vi "raise_any_errors.vi"(8 "error in (no error)":errorcluster, 11 "Request in":refnum<class "Request.lvclass">) -> (0 "error out":errorcluster, 3 "Request out":refnum<class "Request.lvclass">)   [LabVIEW 2020, in "reqwest.lvlib" / "Request.lvclass"]
uses:
  Request.lvclass
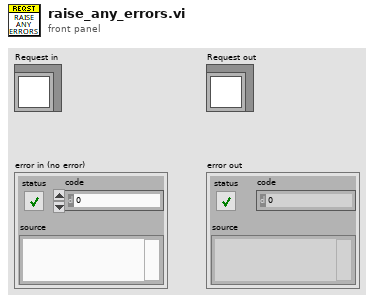
[diagram p1: front panel]
types:
  T1 = typedef "reqwest.lvlib/Request.lvclass/reqwest_error_kind_enum.ctl" = enum16{"none", "timeout", "connection", "redirect", "invalid_status", "body", "decode", "builder", "request", "file_system", "unknown"}
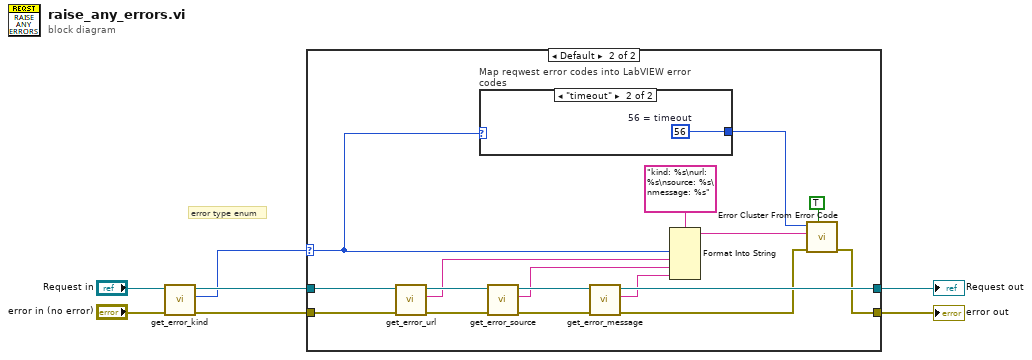
[diagram p0: block diagram]
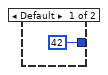
[diagram p3: hidden frame]
diagram:
  # "error type enum"
  n1 = call "get_error_kind.vi"("error in (no error)"="error in (no error)", "Request in"="Request in") -> ("error out"=w2:errorcluster, "error_kind"=w1:T1, "Request out"=w3:refnum<class "Request.lvclass">)  [unwired: 7 in]
  n2 = case shown="Default" w1 {
    selector: w1 -> [_ w10]
    tunnel: [w9 w26] -> w5
    tunnel: [w8 w25] -> w4
    tunnel: w3 -> [w9 w19]
    tunnel: w2 -> [w8 w18]
    frame "none" {
    }
    frame Default {
      n3 = call "get_error_url.vi"("error in (no error)"=w18, "Request in"=w19) -> ("error out"=w16:errorcluster, "error_url"=w15:string, "Request in"=w17:refnum<class "Request.lvclass">)  [unwired: 7 in]
      n4 = case "Map reqwest error codes into LabVIEW error codes" shown="\"timeout\"" w10 {
        tunnel: [42 ("error code (0)") w28] -> w23
        frame Default {
        }
        frame "timeout" {
          w28 = 56  # 56 = timeout
        }
      }
      n5 = call "get_error_source.vi"("error in (no error)"=w16, "Request in"=w17) -> ("error out"=w21:errorcluster, "error_source"=w14:string, "Request in"=w20:refnum<class "Request.lvclass">)  [unwired: 7 in]
      n6 = call "get_error_message.vi"("error in (no error)"=w21, "Request in"=w20) -> ("error out"=w24:errorcluster, "error_message"=w12:string, "Request in"=w26:refnum<class "Request.lvclass">)  [unwired: 7 in]
      n7 = Format Into String(format string="kind: %s\nurl: %s\nsource: %s\nmessage: %s", w10, w15, w14, w12) -> (resulting string=w11:string)  [unwired: 2 in, 1 out]
      n8 = call <vilib>:"Error Cluster From Error Code.vi"("show call chain? (False)"=TRUE, "error in (no error)"=w24, "error message (\"\")"=w11, "error code (0)"=w23) -> ("error out"=w25:errorcluster)  [unwired: 5 in]
    }
  }
  "Request out" <- w5
  "error out" <- w4
